vi "ClosePort.vi"(8 "Uart Input":cluster{u64} {"?" format="%x"}, 11 "Error Input":errorcluster) -> (0 "Uart Output":cluster{u64} {"?" format="%x"}, 3 "Error Output":errorcluster)   [LabVIEW 2019]
doc: "<B>ClosePort</B> the serial port."
uses:
  VC2019/Debug/VIUart.dll
panel:
  # "Close the serial port"
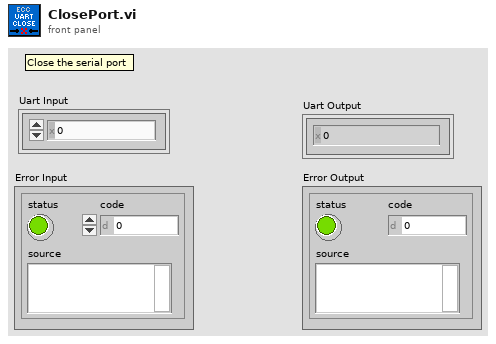
[diagram p1: front panel]
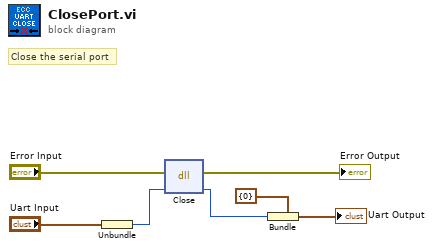
[diagram p0: block diagram]
diagram:
  # "Close the serial port"
  n1 = Unbundle("Uart Input") -> (w4:u64)
  n2 = dll-call lib="C:/Users/drsanti/Desktop/LabVIEW-UART/VC2019/Debug/VIUart.dll" fn="Close"(error in="Error Input", "Uart Handle"=w4) -> (error out=→"Error Output":errorcluster, "Uart Handle"=w1:u64)  [unwired: 3 in, 1 out]
  n3 = Bundle(cluster=cluster{u64} {0}, w1) -> (→"Uart Output":cluster{u64})
